vi "DynamixelMove.vi"(0 "VISA resource name":refnum<visa-resource-name>, 5 "Motor ID (0)":u8, 7 "Goal Position (150 deg)":dbl=150.0, 9 "Goal Speed (RPM)":dbl, 11 "error in (no error)":errorcluster) -> (4 "VISA resource name out":refnum<visa-resource-name>, 15 "error out":errorcluster)   [LabVIEW 2013]
doc: "Sets the goal position or desired velocity for the motor.\nDerived from the library function. However, to make the motors rotate in both directions, we had to change the coercion.\n0-60 scales speed in a linear fashion in the counter clockwise direction. It then remains at the maximum speed until 115, at which point it becomes 0 again. From 115 to 175 it scales in a linear fashion in the clockwise direction. Any greater number remains clockwise at the top speed.\n\n4-7-2014 \nElizabeth Mahon and Eric Schneider"
uses:
  <instrlib>/Dynamixel Motor/Dynamixel Motor.lvlib
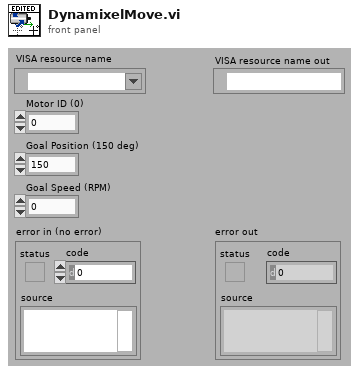
[diagram p1: front panel]
types:
  T1 = enum16{"big-endian, network order", "native, host order", "little-endian"}
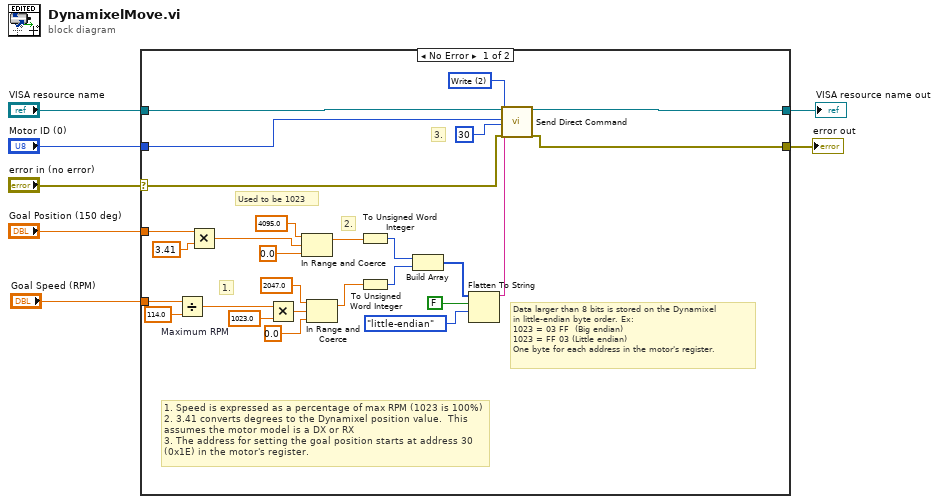
[diagram p0: block diagram]
diagram:
  n1 = case shown="No Error" "error in (no error)" {
    selector: "error in (no error)" -> [w12 w36]
    tunnel: "VISA resource name" -> [w33 w35]
    tunnel: [w32 w35] -> w6
    tunnel: [w31 w36] -> w5
    tunnel: "Motor ID (0)" -> [w30 _]
    tunnel: "Goal Position (150 deg)" -> [w24 _]
    tunnel: "Goal Speed (RPM)" -> [w23 _]
    frame No Error {
      w20 = 114.0  # Maximum RPM
      w34 = u16 2 items=["Ping", "Read", "Write", "Registered Write", "Action", "Reset", "Sync Write"] ("Select Action")
      # "Used to be 1023"
      # "3."
      # "2."
      # "1."
      # "Data larger than 8 bits is stored on the Dynamixel \nin little-endian byte order. Ex:\n1023 = 03 FF  (Big endian)\n1023 = FF 03 (Little endian)\nOne byte for each address in the motor's register."
      # "1. Speed is expressed as a percentage of max RPM (1023 is 100%)\n2. 3.41 converts degrees to the Dynamixel position value.  This \nassumes the motor model is a DX or RX\n3. The address for setting the goal position starts at address 30\n(0x1E) in the motor's register."
      n2 = Divide(x=w23, y=w20) -> (x/y=w22:dbl)
      n3 = Multiply(x=w24, y=3.41) -> (x*y=w8:dbl)
      n4 = Multiply(x=w22, y=1023.0 ("upper limit")) -> (x*y=w27:dbl)
      n5 = In Range and Coerce(upper limit=4095.0, x=w8, lower limit=0.0) -> (coerced(x)=w9:dbl)  [unwired: 1 out]
      n6 = In Range and Coerce(upper limit=2047.0, x=w27, lower limit=0.0) -> (coerced(x)=w14:dbl)  [unwired: 1 out]
      n7 = To Unsigned Word Integer(number=w9) -> (unsigned 16bit integer=w17:u16)
      n8 = To Unsigned Word Integer(number=w14) -> (unsigned 16bit integer=w16:u16)
      n9 = Build Array(w17, w16) -> (w15:u16[])
      n10 = Flatten To String(anything=w15, prepend array or string size? (T)=FALSE, byte order (0:big-endian, network order)=T1."little-endian") -> (data string=w13:string)  [unwired: 1 in, 2 out]
      n11 = call <instrlib>:"Send Direct Command.vi"("VISA resource name"=w33, "Select Action"=w34, "Motor ID (0)"=w30, "Address"=u8 30, "Parameters"=w13, "Error in (no error)"=w12) -> ("VISA resource name out"=w32:refnum<visa-resource-name>, "Error out"=w31:errorcluster)  [unwired: 11 in, 1 out]
    }
    frame Error {
    }
  }
  "VISA resource name out" <- w6
  "error out" <- w5
